vi "add_repeat_measurements_to_queue.vi"(10 "Scan settings array":T3[](array[typedef]) {"J-t settling delay (s)" min=10.0; "J-t illumination" items=["Light only", "Dark only", "Light then dark", "Dark then light"]; "Measurement speed" items=["Fast", "Normal", "High accuracy"]; "Illumination" items=["Light only", "Dark only", "Light then dark", "Dark then light"]; "Only repeat for best pixel" items=["only for best pixel", "for best 2 pixels", "for best 3 pixels", "for best 4 pixels", "for best 5 pixels", "for best 6 pixels", "for best 7 pixels", "for all pixels"]; "No. of repeat scans" min=1.0 step=1.0; "Max power best pixel only" items=["only the best pixel", "the best 2 pixels", "the best 3 pixels", "the best 4 pixels", "the best 5 pixels", "the best 6 pixels", "the best 7 pixels", "all pixels"]; "J-t best pixel only" items=["only the best pixel", "the best 2 pixels", "the best 3 pixels", "the best 4 pixels", "the best 5 pixels", "the best 6 pixels", "the best 7 pixels", "all pixels"]; "J-t measurement speed" items=["Fast", "Normal", "High Accuracy"]; "Stabilisation mode" items=["V", "I"]; "Measurement delay (ms)" min=10.0}, 11 "Cell settings cluster":T2) -> (3 "Repeat light array":T1(array[cluster]))   [LabVIEW 2016]
uses:
  TypeDefs/scan_settings.ctl
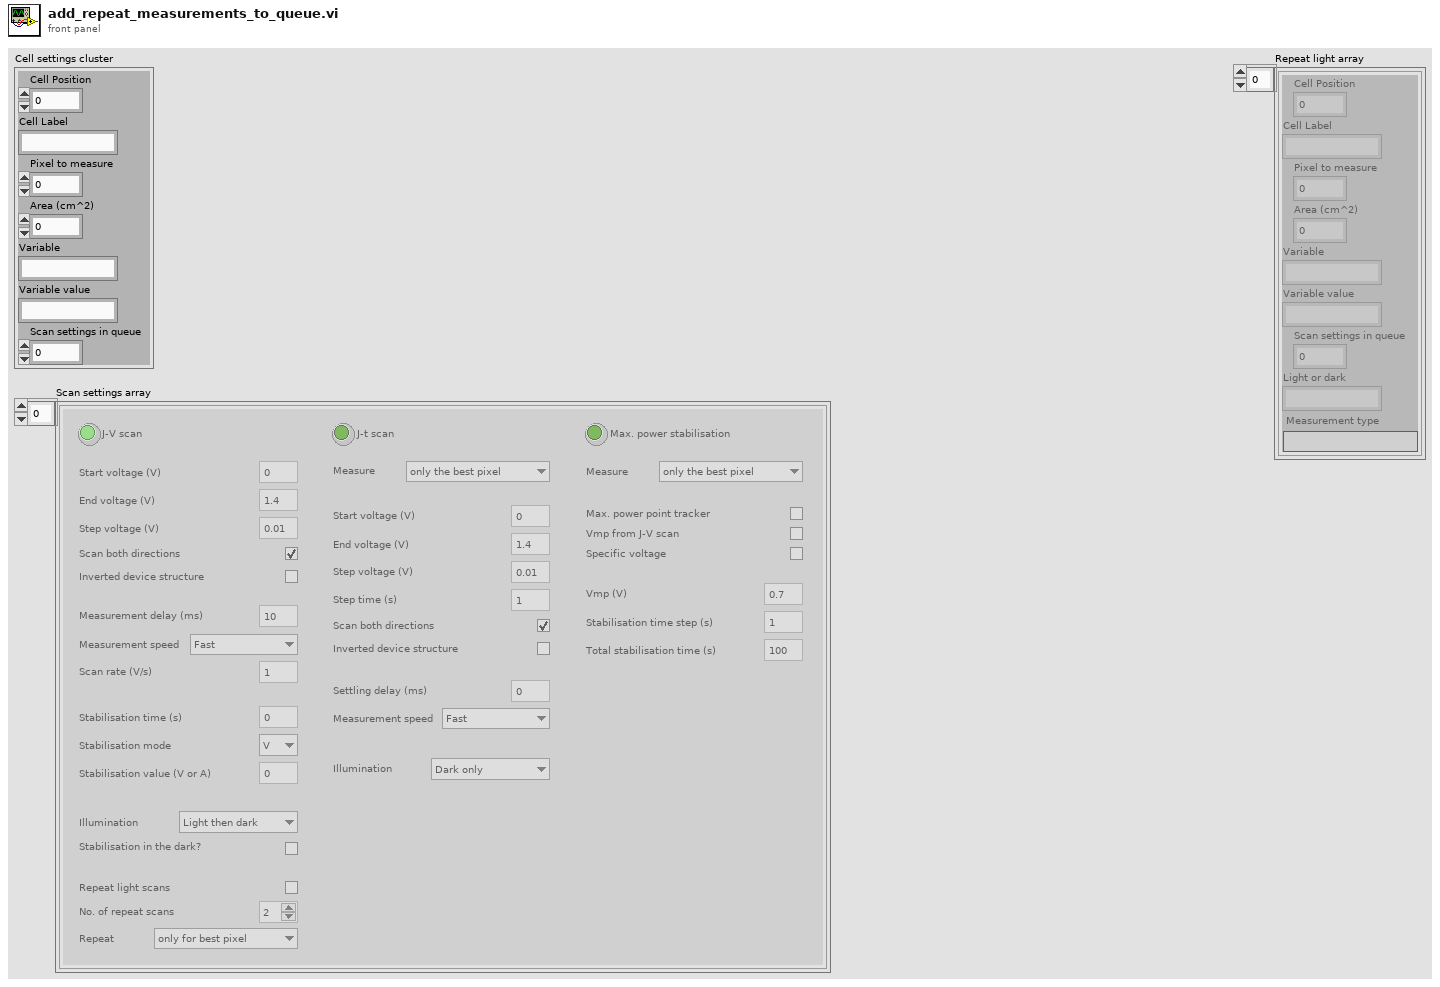
[diagram p1: front panel]
types:
  T1 = cluster{"Cell Position":i32, "Cell Label":string, "Pixel to measure":u16, "Area (cm^2)":dbl, "Variable":string, "Variable value":string, "Scan settings in queue":u16, "Light or dark":string, "Measurement type":string}[]
  T2 = cluster{"Cell Position":i32, "Cell Label":string, "Pixel to measure":u16, "Area (cm^2)":dbl, "Variable":string, "Variable value":string, "Scan settings in queue":u16}
  T3 = typedef "scan_settings.ctl" = cluster{"J-V scan":bool, "Start voltage (V)":dbl, "End voltage (V)":dbl, "Step voltage (V)":dbl, "Scan both directions":bool, "Inverted device structure":bool, "Measurement delay (ms)":dbl, "Measurement speed":u8, "Scan rate (V/s)":dbl, "Stabilisation time (s)":dbl, "Stabilisation mode":u16, "Stabilisation value (V or A) ":dbl, "Illumination":u16, "Stabilisation in the dark?":bool, "Repeat light scans":bool, "No. of repeat scans":dbl, "Only repeat for best pixel":u16, "J-t scan":bool, "J-t best pixel only":u16, "J-t start voltage (V)":dbl, "J-t end voltage (V)":dbl, "J-t step voltage (V)":dbl, "Step time (s)":dbl, "J-t scan both directions":bool, "J-t inverted device structure":bool, "J-t settling delay (s)":dbl, "J-t measurement speed":u16, "J-t illumination":u16, "Max. power stabilisation":bool, "Max power best pixel only":u16, "Max. power point tracker":bool, "Vmp from J-V scan":bool, "Max P stab. Specific voltage":bool, "Vmp (V)":dbl, "Stabilisation time step (s)":dbl, "Total stabilisation time (s)":dbl}
  T4 = cluster{"Cell Position":i32, "Cell Label":string, "Pixel to measure":u16, "Area (cm^2)":dbl, "Variable":string, "Variable value":string, "Scan settings in queue":u16, "Light or dark":string, "Measurement type":string}
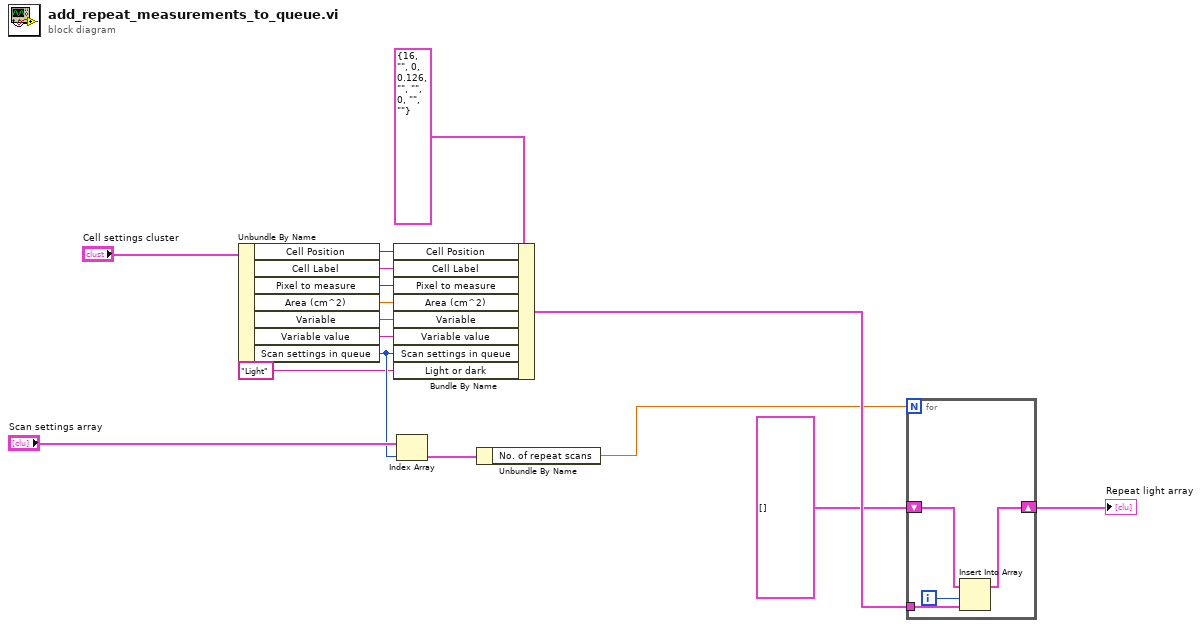
[diagram p0: block diagram]
diagram:
  n1 = Unbundle By Name("Cell settings cluster") -> ("Cell Position"=w5:i32, "Cell Label"=w6:string, "Pixel to measure"=w7:u16, "Area (cm^2)"=w8:dbl, "Variable"=w9:string, "Variable value"=w10:string, "Scan settings in queue"=w14:u16)
  n2 = Bundle By Name(cluster=T4 {"Cell Position"=16, "Cell Label"="", "Pixel to measure"=0, "Area (cm^2)"=0.126, "Variable"="", "Variable value"="", "Scan settings in queue"=0, "Light or dark"="", "Measurement type"=""} ("System Cluster"), "Cell Position"=w5, "Cell Label"=w6, "Pixel to measure"=w7, "Area (cm^2)"=w8, "Variable"=w9, "Variable value"=w10, "Scan settings in queue"=w14, "Light or dark"="Light") -> (w3:T4)
  n3 = Index Array(array="Scan settings array", index=w14) -> (element=w16:T3)
  n4 = Unbundle By Name(w16) -> ("No. of repeat scans"=w2:dbl)
  n5 = for {
    N: w2 -> [_]
    tunnel: w3 -> [w19]
    shift-right: [w17] -> w12
    shift-left: T1 [] ("Light/dark array") -> [w18]
    i -> [w20]
    n6 = Insert Into Array(array=w18, index=w20, new element=w19) -> (w17:T1)
  }
  "Repeat light array" <- w12
